vi "Create Waveform Channel.vi"(8 "error in (no error)":errorcluster, 10 "Bitfile Name":string, 11 "Item Ref in":T1 format="%.0x") -> (0 "error out":errorcluster)   [LabVIEW 2019, in "FPGA Addon System Explorer.lvlib"]
uses:
  FPGA Addon System Explorer.lvlib
  <vilib>/NI VeriStand/Custom Device API/Custom Device Item Ref.ctl
  <vilib>/NI VeriStand/Custom Device API/Custom Device Channel.ctl
  <vilib>/NI VeriStand/Custom Device API/Custom Device Channel Type.ctl
  Addon Shared/SubVIs/Constants.vi
  <vilib>/NI VeriStand/Custom Device API/Custom Device API.lvlib
  Addon Shared/FPGA Addon Shared.lvlib
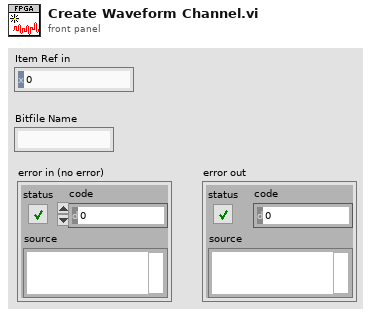
[diagram p1: front panel]
types:
  T1 = typedef "Custom Device API.lvlib/Custom Device Item Ref.ctl" = u64
  T2 = typedef "Custom Device API.lvlib/Custom Device Channel.ctl" = cluster{"Type":T3, "Units":string, "Default Value":dbl, "Faultable":bool, "Scalable":bool}
  T3 = typedef "Custom Device API.lvlib/Custom Device Channel Type.ctl" = enum16{"Input", "Output"}
  T4 = enum32{"invalid app kind", "Development System", "Run Time System", "Student Edition", "Embedded LabVIEW", "Evaluation", "Custom"}
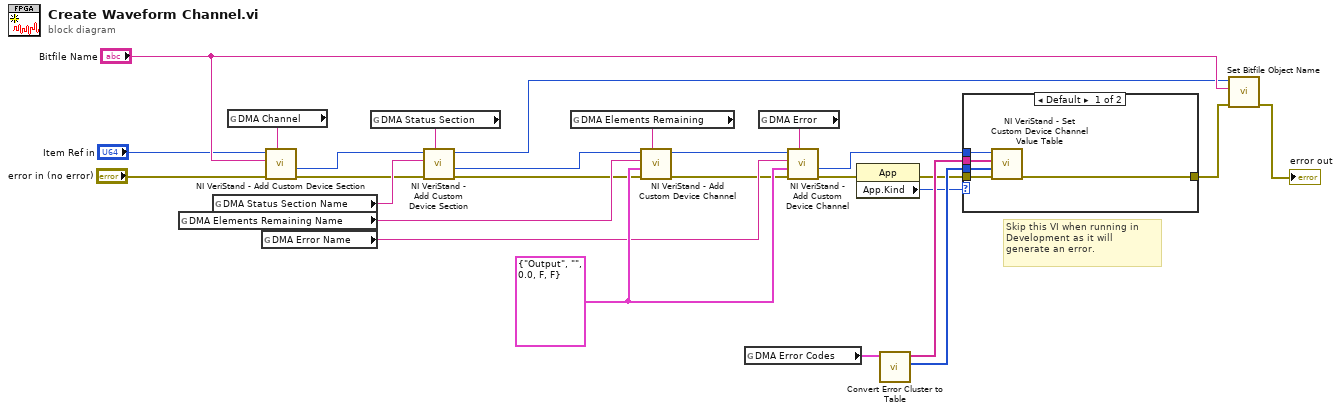
[diagram p0: block diagram]
diagram:
  w17 = T2 {"Type"=enum."Output", "Units"="", "Default Value"=0.0, "Faultable"=FALSE, "Scalable"=FALSE} ("Channel")
  # "Skip this VI when running in Development as it will generate an error."
  n1 = global read "Constants.vi" "DMA Elements Remaining Name"() -> (w14:string)
  n2 = global read "Constants.vi" "DMA Status Section Name"() -> (w18:string)
  n3 = global read "Constants.vi" "DMA Channel"() -> (w6:string)
  n4 = global read "Constants.vi" "DMA Error Name"() -> (w15:string)
  n5 = call <vilib>:"NI VeriStand - Add Custom Device Section.vi"("GUID (Default Section)"=w6, "error in (no error)"="error in (no error)", "Section Name"="Bitfile Name", "Parent Ref in"="Item Ref in") -> ("error out"=w7:errorcluster, "Section Ptr"=w8:T1)  [unwired: 4 in, 2 out]
  n6 = global read "Constants.vi" "DMA Status Section"() -> (w19:string)
  n7 = call <vilib>:"NI VeriStand - Add Custom Device Section.vi"("GUID (Default Section)"=w19, "error in (no error)"=w7, "Section Name"=w18, "Parent Ref in"=w8) -> ("error out"=w12:errorcluster, "Section Ptr"=w11:T1, "Parent Ref out"=w25:T1)  [unwired: 4 in, 1 out]
  n8 = global read "Constants.vi" "DMA Elements Remaining"() -> (w13:string)
  n9 = call <vilib>:"NI VeriStand - Add Custom Device Channel.vi"("GUID (Default Channel)"=w13, "error in (no error)"=w12, "Channel"=w17, "Channel Name"=w14, "Parent Ref in"=w11) -> ("error out"=w10:errorcluster, "Parent Ref out"=w9:T1)  [unwired: 3 in, 2 out]
  n10 = global read "Constants.vi" "DMA Error Codes"() -> (w20:cluster{"number":i32, "trimmed string":string}[])
  n11 = global read "Constants.vi" "DMA Error"() -> (w16:string)
  n12 = call <vilib>:"NI VeriStand - Add Custom Device Channel.vi"("GUID (Default Channel)"=w16, "error in (no error)"=w10, "Channel"=w17, "Channel Name"=w15, "Parent Ref in"=w9) -> ("error out"=w3:errorcluster, "Channel Ref"=w21:T1)  [unwired: 3 in, 2 out]
  n13 = property class="App"(error in=w3) -> (error out=w2:errorcluster, "App.Kind"=w1:T4)  [unwired: 1 in, 1 out]
  n14 = call "Convert Error Cluster to Table.vi"("Error Codes"=w20) -> ("Code"=w23:i32[], "String"=w22:string[])  [unwired: 9 in]
  n15 = case shown="Default" w1 {
    tunnel: [w32 w33] -> w24
    tunnel: w23 -> [w31 _]
    tunnel: w22 -> [w30 _]
    tunnel: w21 -> [w29 _]
    tunnel: w2 -> [w28 w33]
    frame Default {
      n16 = call <vilib>:"NI VeriStand - Set Custom Device Channel Value Table.vi"("error in (no error)"=w28, "Values"=w31, "Names"=w30, "Channel Ref in"=w29) -> ("error out"=w32:errorcluster)  [unwired: 6 in, 1 out]
    }
    frame "Development System" {
    }
  }
  n17 = call "Set Bitfile Object Name.vi"("error in (no error)"=w24, "Name"="Bitfile Name", "Channel Ref"=w25) -> ("error out"=→"error out":errorcluster)  [unwired: 8 in]
